vi "Sets the IR HI SET resistance value for MANU.vi"(5 "Enable to Query":bool, 7 "Enable to Setup":bool, 8 "error in":errorcluster, 9 "IR HI SET resistance value(M£[)":u16=9999 min=2 max=9999, 10 "Sets value to high impedance":u8(ring) items=["High Impedance"=1, "Setup as below"=0], 11 "VISA resource name":refnum<visa-resource-name>) -> (0 "error out":errorcluster, 2 "Return the IR HI SET resistance value":string, 3 "VISA resource name out":refnum<visa-resource-name>)   [LabVIEW 2021, in "GPT-9000.lvlib"]
uses:
  GPT-9000.lvlib
panel:
  # "M£["
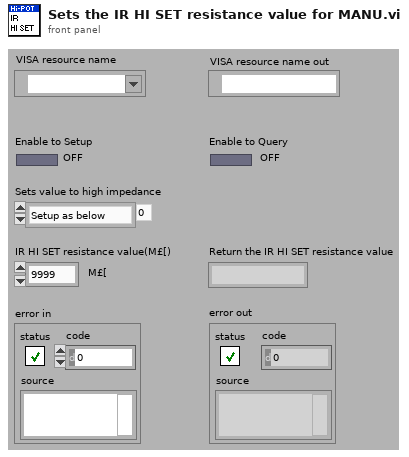
[diagram p1: front panel]
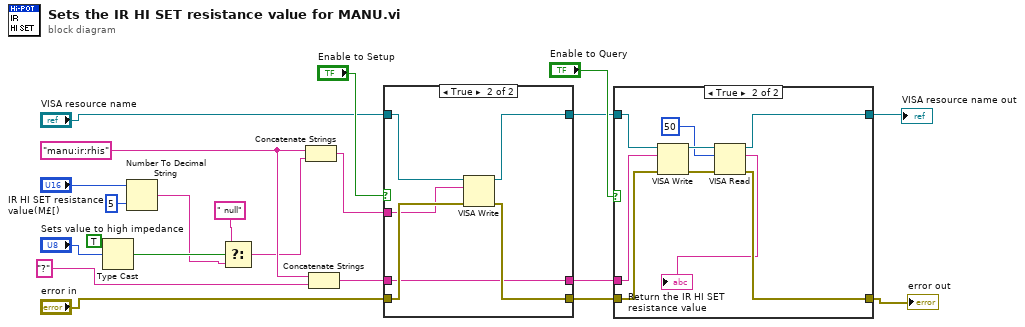
[diagram p0: block diagram]
diagram:
  w21 = "manu:ir:rhis"
  n1 = Type Cast(type=TRUE, x="Sets value to high impedance") -> (*(type *) &x=w4:bool)
  n2 = Number To Decimal String(number="IR HI SET resistance value(M£[)", width (-)=i16 5) -> (decimal integer string=w2:string)
  n3 = Select(t=" null", s=w4, f=w2) -> (s? t:f=w3:string)
  n4 = Concatenate Strings(w21, w3) -> (w19:string)
  n5 = Concatenate Strings(w21, "?") -> (w18:string)
  n6 = case shown="True" "Enable to Setup" {
    tunnel: w19 -> [_ w25]
    tunnel: w18 -> [w22 w26]
    tunnel: "VISA resource name" -> [w24 w30]
    tunnel: "error in" -> [w23 w29]
    tunnel: [w24 w28] -> w14
    tunnel: [w23 w27] -> w13
    tunnel: [w22 w26] -> w12
    frame False {
    }
    frame True {
      n7 = VISA Write(VISA resource name=w30, write buffer=w25, error in (no error)=w29) -> (VISA resource name out=w28:refnum<visa-resource-name>, error out=w27:errorcluster)  [unwired: 1 out]
    }
  }
  n8 = case shown="True" "Enable to Query" {
    tunnel: w14 -> [w32 w40]
    tunnel: w13 -> [w31 w39]
    tunnel: w12 -> [_ w41]
    tunnel: [w32 w35] -> w11
    tunnel: [w31 w34] -> w10
    frame False {
    }
    frame True {
      n9 = VISA Write(VISA resource name=w40, write buffer=w41, error in (no error)=w39) -> (VISA resource name out=w37:refnum<visa-resource-name>, error out=w38:errorcluster)  [unwired: 1 out]
      n10 = VISA Read(VISA resource name=w37, byte count=u32 50, error in (no error)=w38) -> (VISA resource name out=w35:refnum<visa-resource-name>, read buffer=→"Return the IR HI SET resistance value":string, error out=w34:errorcluster)  [unwired: 1 out]
    }
  }
  "VISA resource name out" <- w11
  "error out" <- w10
